vi "ifr2025 Carrier  .vi"(8 "error in (no error)":errorcluster {"code" format="%.0x"}, 11 "instrument handle":refnum<visa-resource-name>) -> (0 "error out":errorcluster {"code" format="%.0x"}, 1 "RF Level":dbl, 2 "Frequency":dbl, 3 "instrument handle out":refnum<visa-resource-name>, 4 "RF Unit":i16, 5 "RF State":i16, 6 "RF Type":i16, 7 "Carrier Mode":i16)   [LabVIEW 2009]
doc: "Returns information about the carrier frequency and RF level of the generator. The units for the returned value of RF level must be specified."
uses:
  Ifr2025_32.dll
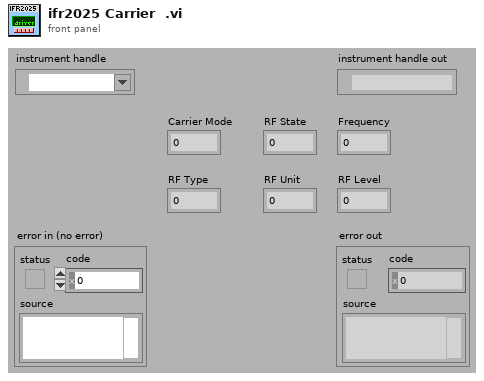
[diagram p1: front panel]
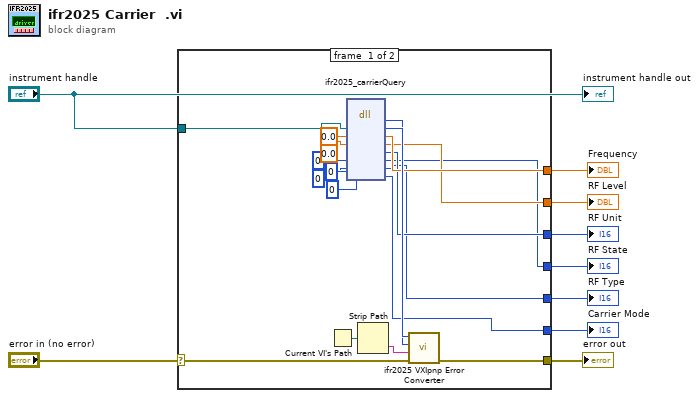
[diagram p0: block diagram]
diagram:
  n1 = case shown="No Error" "error in (no error)" {
    selector: "error in (no error)" -> [w23 w29]
    tunnel: [w22 w29] -> w9
    tunnel: "instrument handle" -> [w27 _]
    tunnel: [w20 _] -> w6
    tunnel: [w18 _] -> w5
    tunnel: [w16 _] -> w4
    tunnel: [w14 _] -> w3
    tunnel: [w12 _] -> w2
    tunnel: [w10 _] -> w1
    frame #0 {
      n2 = Current VI's Path() -> (path=w28:path)
      n3 = dll-call lib="P:/inst/Marconi 2024 Signal Generator/source/labview/ifr2025/ifr2025/ifr2025_*.*" fn="ifr2025_carrierQuery"("vi"=w27, "Frequency"=0.0, "RF Level"=0.0, "RF Unit"=i16 0, "RF State"=i16 0, "RF Type"=i16 0, "Carrier Mode"=i16 0) -> (w25:i32, "vi"=w26:u32, "Frequency"=w20:dbl, "RF Level"=w18:dbl, "RF Unit"=w16:i16, "RF State"=w14:i16, "RF Type"=w12:i16, "Carrier Mode"=w10:i16)  [unwired: 3 in, 2 out]
      n4 = Strip Path(path=w28) -> (name=w24:string)  [unwired: 1 out]
      n5 = call "ifr2025 VXIpnp Error Converter.vi"("error in (no error)"=w23, "name of VI (\"\")"=w24, "CVI error code (0)"=w25, "instrument handle"=w26) -> ("error out"=w22:errorcluster)  [unwired: 7 out]
    }
    frame #1 {
    }
  }
  "error out" <- w9
  "Frequency" <- w6
  "RF Level" <- w5
  "RF Unit" <- w4
  "RF State" <- w3
  "RF Type" <- w2
  "Carrier Mode" <- w1
  "instrument handle out" <- "instrument handle"
